vi "Encoder Lift.vi"(11 "Inches":dbl) -> ()   [LabVIEW 2014]
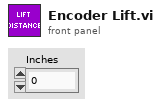
[diagram p1: front panel]
types:
  T1 = typedef "WPI_EncoderDevRef.ctl" = cluster{"DevStatus":errorcluster, "EncoderIndex":T2, "CounterIndex":T3, "DistancePerCount":dbl, "Decoding Type":T4}
  T2 = typedef "FPGA_EncoderIdx.ctl" = enum8{"Enc 0", "Enc 1", "Enc 2", "Enc 3", "Enc 4", "Enc 5", "Enc 6", "Enc 7", "Invalid"}
  T3 = typedef "FPGA_CounterCtrSystemIndex.ctl" = enum8{"Ctr 0", "Ctr 1", "Ctr 2", "Ctr 3", "Ctr 4", "Ctr 5", "Ctr 6", "Ctr 7", "Invalid"}
  T4 = typedef "WPI_EncoderType.ctl" = enum16{"1x", "2x", "4x"}
  T5 = typedef "WPI_MotorControlDeviceRef.ctl" = cluster{"DeviceStatus":errorcluster, "Type":T6, "PWM":cluster{"Controller":T7, "PWM Channel":T8, "DeadBand":T9}, "CAN":cluster{"Device Number":u8, "Control Mode":T10, "Semaphore":T11, "Max Vout":dbl, "TalonSRX Control Mode":T12}, "Invert":bool, "TransformRef":T13, "InvTransformRef":T13}
  T6 = typedef "WPI_MotorControlType.ctl" = enum16{"PWM", "CAN", "CANTalonSRX"}
  T7 = typedef "FPGA_TypedefDigitalModule.ctl" = enum16{"Controller 1"}
  T8 = typedef "FPGA_DIOPWMChannel.ctl" = enum8{"PWM 0", "PWM 1", "PWM 2", "PWM 3", "PWM 4", "PWM 5", "PWM 6", "PWM 7", "PWM 8", "PWM 9", "PWM MXP 0", "PWM MXP 1", "PWM MXP 2", "PWM MXP 3", "PWM MXP 4", "PWM MXP 5", "PWM MXP 6", "PWM MXP 7", "PWM MXP 8", "PWM MXP 9", "Invalid"}
  T9 = typedef "WPI_PWMDeadband.ctl" = cluster{"Name":string, "maxPositivePwm":i32, "minPositivePwm":i32, "centerPwm":i32, "maxNegativePwm":i32, "minNegativePwm":i32, "angularRange":u16}
  T10 = typedef "WPI_CANJaguar_ControlMode.ctl" = enum8{"Percent VBus", "Current", "Speed", "Position", "Voltage"}
  T11 = typedef "Semaphore RefNum" = refnum<k1>
  T12 = typedef "WPI_CANTalonSRX_APIControlMode.ctl" = enum8{"Percent VBus", "Speed", "Position", "Slave", "Unchanged / Invalid"}
  T13 = typedef "WPI_PWMTransform_ConPane.ctl" = refnum<vi>
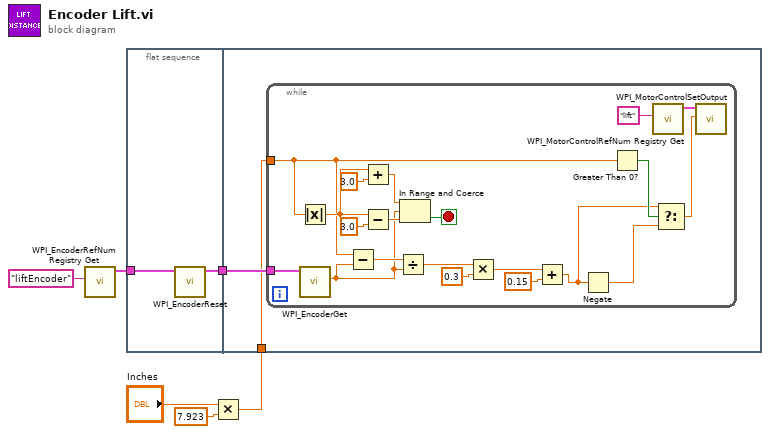
[diagram p0: block diagram]
diagram:
  n1 = call <vilib>:"WPI_EncoderRefNum Registry Get.vi"("refnum name"="liftEncoder") -> ("EncoderDevRef"=w6:T1)  [unwired: 9 in, 1 out]
  n2 = flat-sequence {
    tunnel: w6 -> [w8]
    tunnel: [w7] -> w5
    tunnel: w5 -> [w10]
    tunnel: w1 -> [w9]
    frame #0 {
      n3 = call <vilib>:"WPI_EncoderReset.vi"("EncoderDevRef"=w8) -> ("EncoderDevRef"=w7:T1)  [unwired: 9 in, 1 out]
    }
    frame #1 {
      n4 = while {
        tunnel: w10 -> [w30]
        tunnel: w9 -> [w22]
        stop <- w23 stop-if-true
        n5 = Absolute Value(x=w22) -> (abs(x)=w26:dbl)
        n6 = call <vilib>:"WPI_EncoderGet.vi"("EncoderDevRef"=w30) -> ("Distance"=w20:dbl)  [unwired: 5 in, 5 out]
        n7 = Subtract(x=w22, y=w20) -> (x-y=w21:dbl)
        n8 = Add(x=w26, y=3.0) -> (x+y=w24:dbl)
        n9 = Subtract(x=w26, y=3.0) -> (x-y=w27:dbl)
        n10 = Divide(x=w21, y=w20) -> (x/y=w19:dbl)
        n11 = In Range and Coerce(upper limit=w24, x=w20, lower limit=w27) -> (In Range?=w23:bool)  [unwired: 1 out]
        n12 = Multiply(x=w19, y=0.3) -> (x*y=w17:dbl)
        n13 = Add(x=w17, y=0.15 ("x*y")) -> (x+y=w11:dbl)
        n14 = Negate(x=w11) -> (-x=w15:dbl)
        n15 = Greater Than 0?(x=w22) -> (x > 0?=w29:bool)
        n16 = call <vilib>:"WPI_MotorControlRefNum Registry Get.vi"("refnum name"="lift") -> ("MotorControlDevRef"=w14:T5)  [unwired: 9 in, 1 out]
        n17 = Select(t=w11, s=w29, f=w15) -> (s? t:f=w12:dbl)
        n18 = call <vilib>:"WPI_MotorControlSetOutput.vi"("Output"=w12, "MotorControlDevRef"=w14) -> ()  [unwired: 7 in, 3 out]
      }
    }
  }
  n19 = Multiply(x="Inches", y=7.923) -> (x*y=w1:dbl)
